vi "update counter entry.vi"   [LabVIEW 2015]
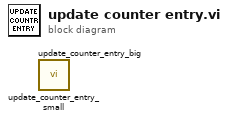
[diagram p0: block diagram]
diagram:
  n1 = call "update_counter_entry_small.vi"() -> ()  [unwired: 11 in, 1 out]
  n2 = call "update_counter_entry_big.vi"() -> ()  [unwired: 11 in, 1 out]
